vi "CALC_MARK_STAT_ON_OFF.vi"(0 "VISA IN":refnum<visa-resource-name>, 1 "Marker number":u16, 2 "Marker ON/OFF":bool, 5 "error in":errorcluster, 7 "Channel":i32) -> (14 "VISA Out":refnum<visa-resource-name>, 19 "error out":errorcluster)   [LabVIEW 2018, in "PNA-X.lvlib"]
doc: "CALCulate<cnum>:MARKer<mkr>[:STATe] <ON|OFF> \n1541\n\n(Read-Write) Turns the specified marker ON or OFF. Marker 10 is the Reference Marker. To turn \nall markers off, use CALC:MARK:AOFF. \nSee Critical Note \nParameters \n<cnum> Channel number of the measurement. There must be a selected measurement \non that channel. If unspecified, <cnum> is set to 1. \n<mkr> Any marker number from 1 to 10; if unspecified, value is set to 1. \n<ON|OFF> ON (or 1) - turns marker ON. \nOFF (or 0) - turns marker OFF. \nExamples CALC:MARK ON \ncalculate2:marker8 on \nQuery Syntax CALCulate<cnum>:MARKer<mkr>:STATe? \nReturn Type Boolean (1 = ON, 0 = OFF) \nDefault Off"
uses:
  PNA-X.lvlib
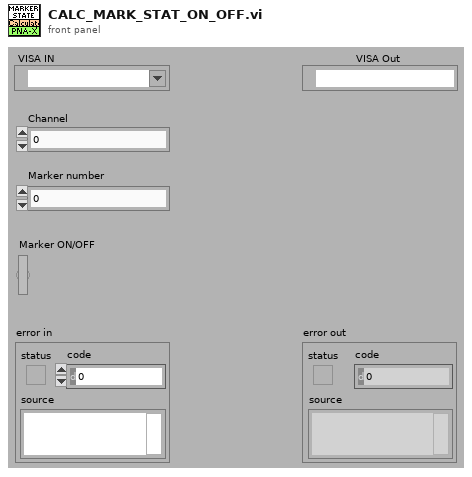
[diagram p1: front panel]
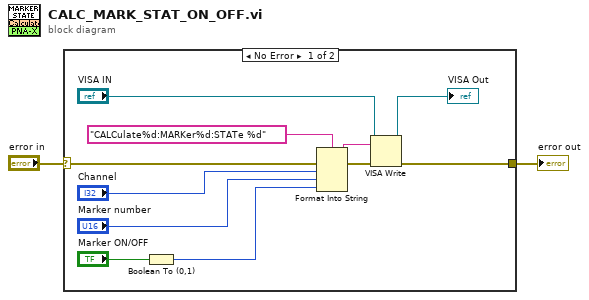
[diagram p0: block diagram]
diagram:
  n1 = case shown="No Error" "error in" {
    selector: "error in" -> [w13 w14]
    tunnel: [w8 w14] -> w1
    frame No Error {
      n2 = Boolean To (0,1)(Boolean="Marker ON/OFF") -> (0, 1=w3:i16)
      n3 = Format Into String(format string="CALCulate%d:MARKer%d:STATe %d" ("Cmdline"), error in=w13, "Channel", "Marker number", w3) -> (resulting string=w11:string, error out=w12:errorcluster)  [unwired: 1 in]
      n4 = VISA Write(VISA resource name="VISA IN", write buffer=w11, error in (no error)=w12) -> (VISA resource name out=→"VISA Out":refnum<visa-resource-name>, error out=w8:errorcluster)  [unwired: 1 out]
    }
    frame Error {
    }
  }
  "error out" <- w1
